vi "Write to Command Line.vi"(6 "LF":bool=TRUE caption="Append End-Line (T)", 8 "error in (no error)":errorcluster, 10 "Message":string, 11 "Builder in":refnum<class "Builder.lvclass">) -> (0 "error out":errorcluster, 3 "Builder out":refnum<class "Builder.lvclass">)   [LabVIEW 2019, in "Builder.lvclass"]
uses:
  Builder.lvclass
  Builder.lvclass/Builder.ctl
  CLI Output/CLI Output.lvclass
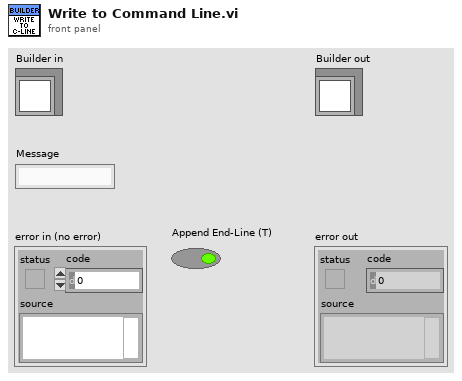
[diagram p1: front panel]
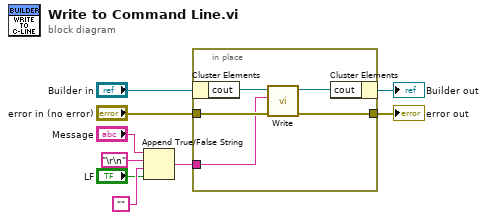
[diagram p0: block diagram]
diagram:
  n1 = Append True/False String(1:"LF", 2:"", 3:"\r\n", 4:"Message") -> (0:w3:string)
  n2 = in-place {
    in-place-border: "error in (no error)" -> [w12]
    in-place-border: [w11] -> w5
    in-place-border: w3 -> [w10]
    n3 = in-place-cluster #1("Builder in") -> ("cout"=w14:refnum<class "CLI Output.lvclass">)
    n4 = call-dynamic "Write.vi"("error in (no error)"=w12, "String"=w10, "CLI Output in"=w14) -> ("error out"=w11:errorcluster, "CLI Output out"=w13:refnum<class "CLI Output.lvclass">)  [unwired: 7 in]
    n5 = in-place-cluster #1("cout"=w13) -> (→"Builder out":refnum<class "Builder.lvclass">)
  }
  "error out" <- w5
